vi "ma.vi"(1 "c":u32, 2 "b":u32, 3 "a":u32) -> (0 "ma":u32)   [LabVIEW 2019, in "SHA256.lvlib"]
doc: "Calculates the ma variable in the schedule compression phase"
uses:
  Downloads/LabVIEW-Bits-master-2/Cryptographic Services/SHA256/SHA256.lvlib
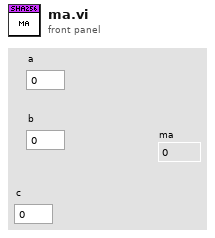
[diagram p1: front panel]
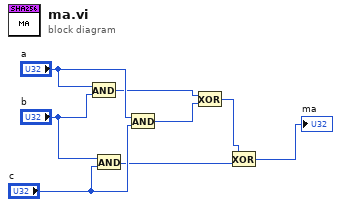
[diagram p0: block diagram]
diagram:
  n1 = And(x="a", y="b") -> (x .and. y?=w5:u32)
  n2 = And(x="b", y="c") -> (x .and. y?=w2:u32)
  n3 = And(x="a", y="c") -> (x .and. y?=w4:u32)
  n4 = Exclusive Or(1:w4, 2:w5) -> (0:w3:u32)
  n5 = Exclusive Or(1:w2, 2:w3) -> (0:→"ma":u32)
